vi "M Water Cells.vi"(11 "EV3 in":T1) -> ()   [LabVIEW 2016]
uses:
  <vilib>/NXT/Subs/LVHSConnector.ctl
  <vilib>/NXT/LegoClasses/BrickReference/BrickReference.lvclass
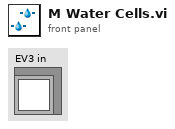
[diagram p1: front panel]
types:
  T1 = typedef "LVHSConnector.ctl" = refnum<class "BrickReference.lvclass">
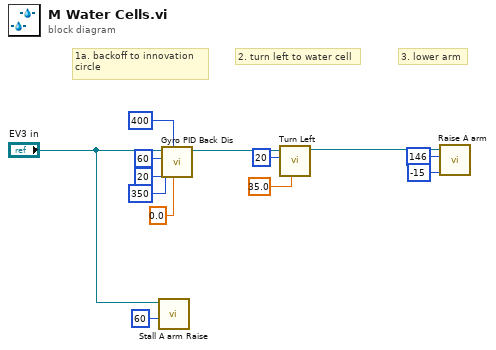
[diagram p0: block diagram]
diagram:
  # "3. lower arm"
  # "2. turn left to water cell"
  # "1a. backoff to innovation\ncircle"
  n1 = call "Stall A arm Raise.vi"("Power"=i8 60, "NXT/EV3"="EV3 in") -> ()  [unwired: 9 in, 1 out]
  n2 = call "Gyro PID Back Dis.vi"("Target angle"=sgl 0.0, "Threshold to stop"=400, "Threshold to slow"=350, "Min. speed"=20, "Max. speed"=60, "EV3 in"="EV3 in") -> ("EV3 out"=w8:T1)  [unwired: 5 in]
  n3 = call "Turn Left.vi"("Turning angle"=sgl 35.0, "Motor B (right)"=i8 20, "EV3 in"=w8) -> ("EV3 out"=w5:T1)  [unwired: 8 in]
  n4 = call "Raise A arm.vi"("Power"=i8 -15, "Rotation"=146, "EV3 in"=w5) -> ()  [unwired: 8 in, 1 out]
